vi "_activate.vi"(8 "error in (no error)":errorcluster, 10 "a_pDeviceId IN":u8[](array[numeric]), 11 "UV-VIS_AVANTES in":refnum<class "UV-VIS_AVANTES.lvclass">) -> (0 "error out":errorcluster, 3 "UV-VIS_AVANTES out":refnum<class "UV-VIS_AVANTES.lvclass">)   [LabVIEW 2020, in "UV-VIS_AVANTES.lvclass"]
uses:
  UV-VIS_AVANTES.lvclass
  C:/dev/TRANCON/Classes/Detector/Detector.lvclass
  Detector.lvclass/Detector.ctl
  UV-VIS_AVANTES.lvclass/UV-VIS_AVANTES.ctl
  Detector.lvclass
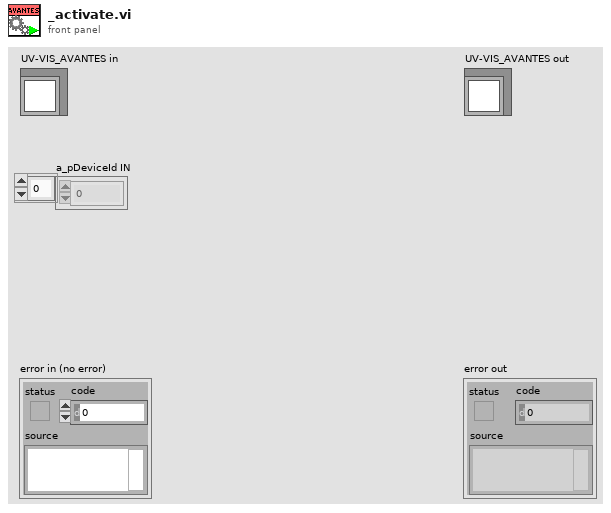
[diagram p1: front panel]
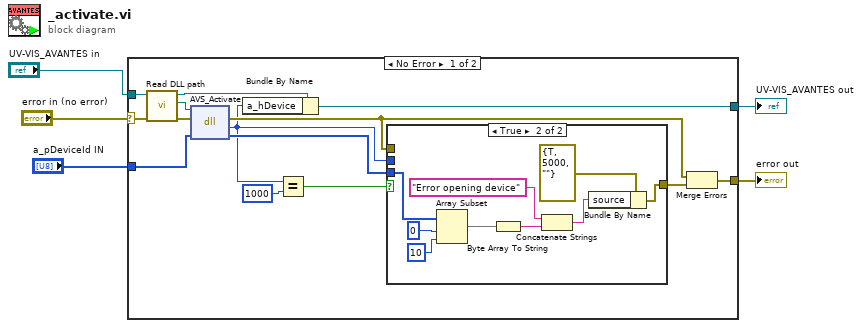
[diagram p0: block diagram]
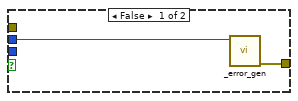
[diagram p2: hidden frame]
diagram:
  n1 = case shown="No Error" "error in (no error)" {
    selector: "error in (no error)" -> [w18 w32]
    tunnel: [w7 w32] -> w4
    tunnel: [w10 w31] -> w2
    tunnel: "UV-VIS_AVANTES in" -> [w19 w31]
    tunnel: "a_pDeviceId IN" -> [w12 _]
    frame No Error {
      n2 = call "Read DLL path.vi"("error in (no error)"=w18, "Detector in"=w19) -> ("error out"=w16:errorcluster, "DLL path"=w17:path, "Detector out"=w11:refnum<class "UV-VIS_AVANTES.lvclass">)  [unwired: 7 in]
      n3 = dll-call lib="C:/AvaSpecX64-DLL_9.4/examples/LabView/LabViewSingleChan/avaspec.dll" fn="AVS_Activate"(path in=w17, error in=w16, "a_pDeviceId"=w12) -> (error out=w9:errorcluster, "return type"=w6:i32, "a_pDeviceId"=w13:u8[])  [unwired: 1 in, 1 out]
      n4 = Bundle By Name(cluster=w11, "a_hDevice"=w6) -> (w10:refnum<class "UV-VIS_AVANTES.lvclass">)
      n5 = Equal?(x=w6, y=1000) -> (x = y?=w14:bool)
      n6 = case shown="True" w14 {
        tunnel: w13 -> [_ w25]
        tunnel: [w21 w22] -> w8
        tunnel: w9 -> [_ _]
        tunnel: w6 -> [w20 _]
        frame False {
          n7 = call "_error_gen.vi"("return type"=w20) -> ("error out"=w21:errorcluster)  [unwired: 10 in]
        }
        frame True {
          n8 = Array Subset(array=w25, index=0 ("length"), length=10) -> (w26:u8[])
          n9 = Byte Array To String(unsigned byte array=w26) -> (string=w28:string)
          n10 = Concatenate Strings("Error opening device", w28) -> (w23:string)
          n11 = Bundle By Name(cluster=errorcluster {"status"=TRUE, "code"=5000, "source"=""} ("error constant"), "source"=w23) -> (w22:errorcluster)
        }
      }
      n12 = Merge Errors(w9, w8) -> (w7:errorcluster)
    }
    frame Error {
    }
  }
  "error out" <- w4
  "UV-VIS_AVANTES out" <- w2
